vi "Relative time.vi"(2 "MASTER in":T1 {"Image data"."Color Palette" items=["Grayscale U8", "False Color", "Overexposed"]; "Image data"."Exposure time [us]" format="%#_10g"; "Queue"."Initial time [s]" format="%_19f"; "Queue"."Raw data [V]\n(all samples)" format="%0.2f"; "Queue"."Timestamp [s]" format="%_19f"}, 7 "Initial time in":dbl format="%_19f") -> (1 "Timestamp":dbl, 4 "Initial time out":dbl format="%_19f", 6 "MASTER out":T1 {"Image data"."Color Palette" items=["Grayscale U8", "False Color", "Overexposed"]; "Image data"."Exposure time [us]" format="%#_10g"; "Queue"."Initial time [s]" format="%_19f"; "Queue"."Raw data [V]\n(all samples)" format="%0.2f"; "Queue"."Timestamp [s]" format="%_19f"})   [LabVIEW 2020]
uses:
  MASTER.ctl
  Constants.ctl
  QBundle.ctl
  Queue.ctl
  Image data.ctl
  <vilib>/userdefined/High Color/IMAQdx.ctl
  <vilib>/vision/Image Controls.llb/IMAQ Image.ctl
  Image QBundle.ctl
panel:
  # "Description:\n\"Absolute time\" mode sets the timestamp to the current time. \"Relative time\" mode subtracts the initial time from the current time to determine the relative timestamp from when the record control was switched on."
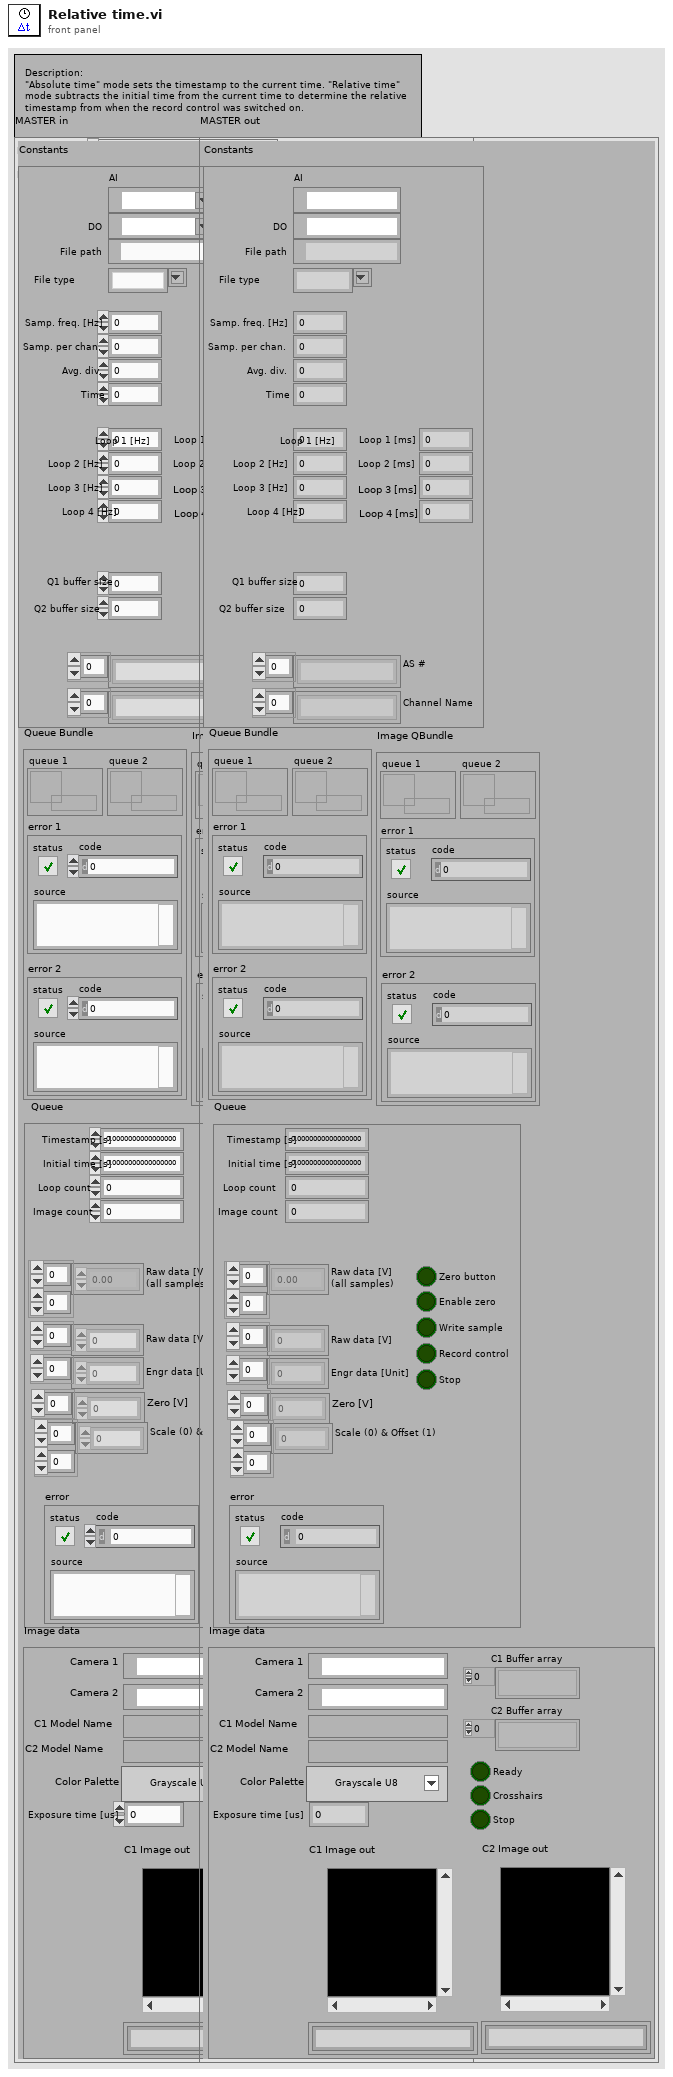
[diagram p1: front panel]
types:
  T1 = typedef "MASTER.ctl" = cluster{"Constants":T2, "Queue Bundle":T3, "Queue":T4, "Image data":T5, "Image QBundle ":T8}
  T2 = typedef "Constants.ctl" = cluster{"Time":u16, "Samp. freq. [Hz]":dbl, "Samp. per chan.":i32, "Avg. div.":i32, "File path":path, "AI":refnum<k21>, "Loop 1 [Hz]":dbl, "Loop 2 [Hz]":dbl, "Loop 3 [Hz]":dbl, "Loop 1 [ms]":dbl, "Loop 2 [ms]":dbl, "Loop 3 [ms]":dbl, "Q1 buffer size":i32, "Q2 buffer size":i32, "File type":string, "Loop 4 [Hz]":dbl, "Loop 4 [ms]":dbl, "Channel Name":string[], "AS #":string[], "DO":refnum<k21>}
  T3 = typedef "QBundle.ctl" = cluster{"queue 1":refnum<queue>, "error 1":errorcluster, "queue 2":refnum<queue>, "error 2":errorcluster}
  T4 = typedef "Queue.ctl" = cluster{"Enable zero":bool, "Engr data [Unit]":dbl[], "Zero button":bool, "Zero [V]":dbl[], "Timestamp [s]":dbl, "Write sample":bool, "Record control":bool, "Stop":bool, "error":errorcluster, "Raw data [V]\n(all samples)":dbl[][], "Raw data [V]":dbl[], "Loop count":i64, "Initial time [s]":dbl, "Scale (0) & Offset (1)":dbl[][], "Image count":dbl}
  T5 = typedef "Image data.ctl" = cluster{"Camera 1":T6, "Camera 2":T6, "C1 Image out ":T7, "C2 Image out":T7, "C1 Model Name":string, "C2 Model Name":string, "Exposure time [us]":dbl, "Color Palette":u16, "C1 Buffer array":T7[], "Ready":bool, "C2 Buffer array":T7[], "Crosshairs":bool, "Stop":bool}
  T6 = typedef "IMAQdx.ctl" = refnum<k21>
  T7 = typedef "IMAQ Image.ctl" = refnum<image>
  T8 = typedef "Image QBundle.ctl" = cluster{"queue 1":refnum<queue>, "error 1":errorcluster, "queue 2":refnum<queue>, "error 2":errorcluster}
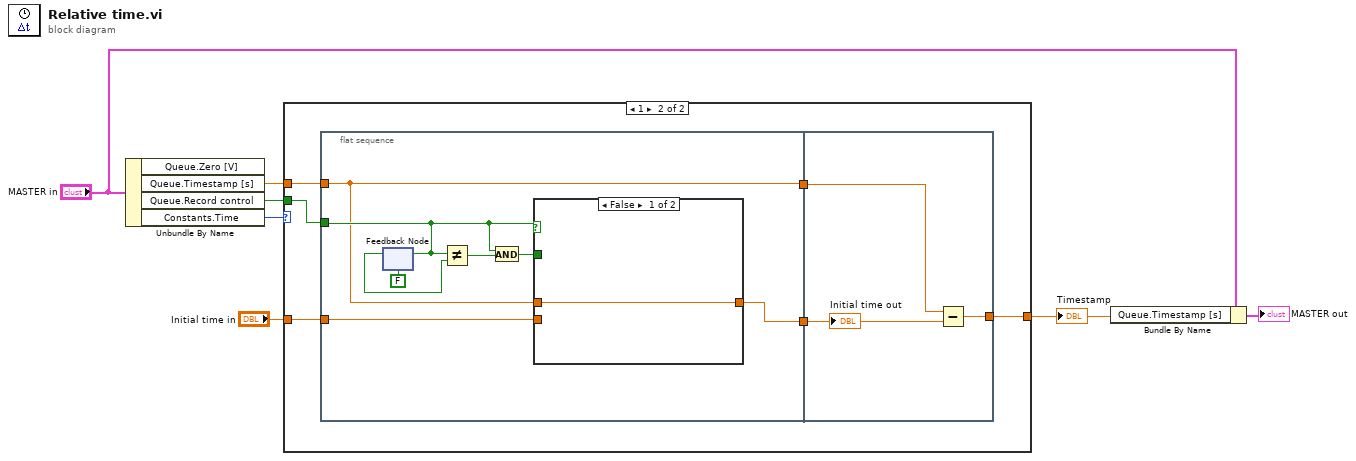
[diagram p0: block diagram]
diagram:
  n1 = Unbundle By Name("MASTER in") -> ("Queue.Timestamp [s]"=w5:dbl, "Queue.Record control"=w7:bool, "Constants.Time"=w2:u16)  [unwired: 1 out]
  n2 = case shown="1" w2 {
    tunnel: "Initial time in" -> [_ w14]
    tunnel: w5 -> [w8 w13]
    tunnel: w7 -> [_ w12]
    tunnel: [w8 w11] -> w6
    frame 0, Default {
    }
    frame 1 {
      n3 = flat-sequence {
        tunnel: w14 -> [w18]
        tunnel: w13 -> [w16]
        tunnel: w12 -> [w17]
        tunnel: [w16] -> w10
        tunnel: [w15] -> w9
        tunnel: [w32] -> w11
        tunnel: w10 -> [w31]
        tunnel: w9 -> [w30]
        frame #0 {
          n4 = feedback #1(FALSE ("Record control")) -> (w22:bool)
          n5 = feedback-in #1(w17) -> ()
          n6 = Not Equal?(x=w17, y=w22) -> (x != y?=w20:bool)
          n7 = And(x=w17, y=w20) -> (x .and. y?=w19:bool)
          n8 = case shown="False" w17 {
            tunnel: w16 -> [w23 w27]
            tunnel: w19 -> [_ w26]
            tunnel: w18 -> [_ w25]
            tunnel: [w23 w24] -> w15
            frame False {
            }
            frame True {
              n9 = case shown="False" w26 {
                tunnel: w27 -> [_ w29]
                tunnel: w25 -> [w28 _]
                tunnel: [w28 w29] -> w24
                frame False {
                }
                frame True {
                }
              }
            }
          }
        }
        frame #1 {
          n10 = Subtract(x=w31, y=w30) -> (x-y=w32:dbl)
          "Initial time out" <- w30
        }
      }
    }
  }
  "Timestamp" <- w6
  n11 = Bundle By Name(cluster="MASTER in", "Queue.Timestamp [s]"=w6) -> (→"MASTER out":T1)
